vi "AudioTest.Play_Record.vi"(6 "Record Device ID":u32, 7 "Play Device ID":u32=1, 8 "error in (no error)":errorcluster, 9 "Sample Rate (Hz)":dbl, 10 "volume":dbl=40.0 format="%#_13g", 11 "Stimulus Wvfrm":waveform(dbl)(graph)) -> (0 "Error Out":errorcluster, 2 "PlayDur(s)":dbl=1.0 format="%.2p", 3 "Recorded Wvfrm":waveform(dbl)(graph))   [LabVIEW 2018]
uses:
  <vilib>/sound2/lvsound2.llb/Sampling Mode.ctl
  <vilib>/sound2/lvsound2.llb/Sound Data Format.ctl
  Common/Utils/Errors/Error.Error Code List.ctl
  <vilib>/sound2/lvsound2.llb/Sound Output Set Volume (Single).vi
  <vilib>/sound2/lvsound2.llb/Sound Output Write (DBL Single).vi
  <vilib>/sound2/lvsound2.llb/Sound Input Read (DBL).vi
panel:
  in  "Pad Time(s)":dbl=0.25 format="%#_13g"
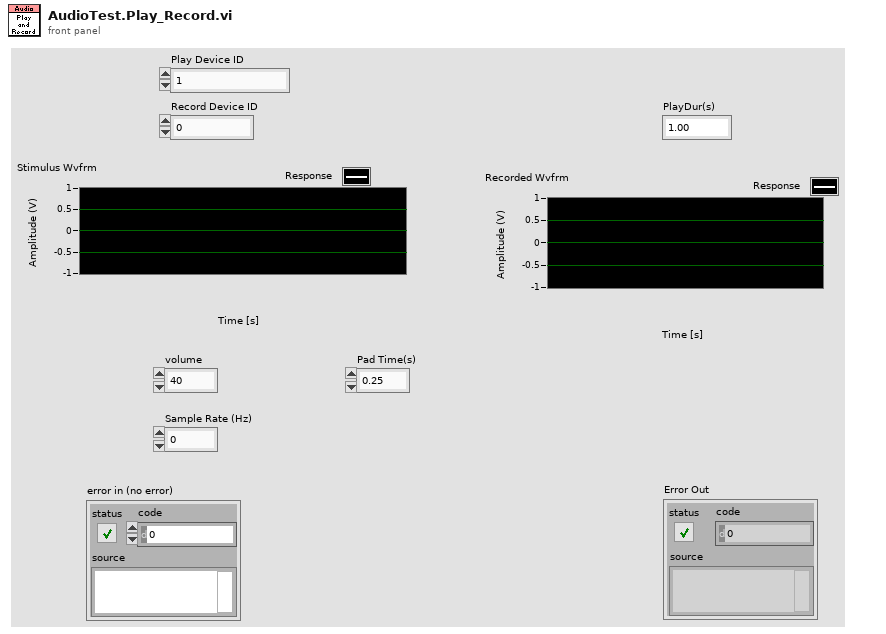
[diagram p1: front panel]
types:
  T1 = typedef "Sound Data Format.ctl" = cluster{"sample rate (S/s)":dbl, "number of channels":i32, "bits per sample":i32}
  T2 = typedef "Error.Error Code List.ctl" = i32
  T3 = typedef "Sampling Mode.ctl" = i32
  T4 = typedef "Sound Output Task ID.ctl" = u32
  T5 = typedef "Sound Input Task ID.ctl" = u32
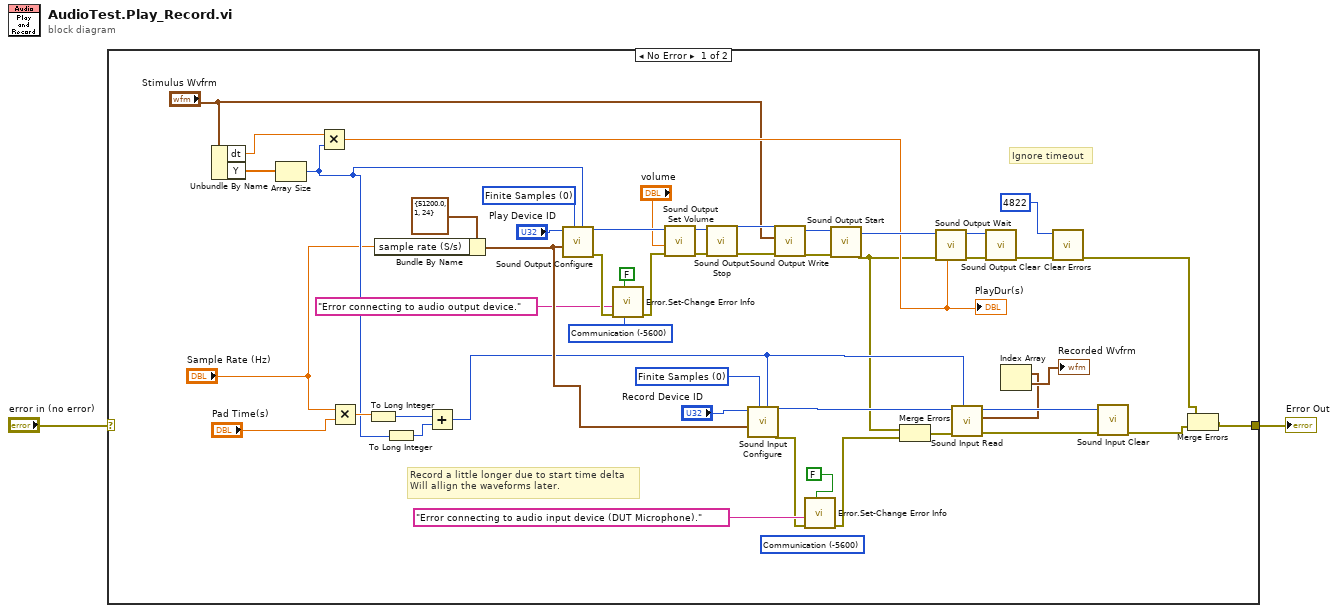
[diagram p0: block diagram]
diagram:
  n1 = case shown="No Error" "error in (no error)" {
    selector: "error in (no error)" -> [_ w52]
    tunnel: [w12 w52] -> w2
    frame No Error {
      (unwired) T2 -5600 items=["No Error"=0, "Abort"=-2, "Misc"=-5000, "Fixture Error"=-5100, "File IO - General"=-5200, "FIle IO - Config Error"=-5201, "Instrument - General"=-5300, "Instrument - Serial Com"=-5301, "Instrument - Camera"=-5302, "Instrument - PS"=-5303, "Instrument - Oscilloscope"=-5304, "Instrument - Function Gen"=-5305, "Instrument - Load"=-5306, "Instrument - Meter"=-5307, "Instrument - Power Control"=-5308, "Instrument - Motion"=-5309, "Instrument - RF"=-5310, "System Exe"=-5400, "Image Processing"=-5500, "Communication"=-5600, "Script - Syntax Error"=-6000, "Script - Invalid Name or Param"=-6100, "Script - Timeout"=-6200, "Invalid Data"=-6300, "FW Update Error"=-6500] ("Std Code")
      w9 = T2 -5600 items=["No Error"=0, "Abort"=-2, "Misc"=-5000, "Fixture Error"=-5100, "File IO - General"=-5200, "FIle IO - Config Error"=-5201, "Instrument - General"=-5300, "Instrument - Serial Com"=-5301, "Instrument - Camera"=-5302, "Instrument - PS"=-5303, "Instrument - Oscilloscope"=-5304, "Instrument - Function Gen"=-5305, "Instrument - Load"=-5306, "Instrument - Meter"=-5307, "Instrument - Power Control"=-5308, "Instrument - Motion"=-5309, "Instrument - RF"=-5310, "System Exe"=-5400, "Image Processing"=-5500, "Communication"=-5600, "Script - Syntax Error"=-6000, "Script - Invalid Name or Param"=-6100, "Script - Timeout"=-6200, "Invalid Data"=-6300, "FW Update Error"=-6500] ("Std Code")
      w46 = T3 0 items=["Finite Samples", "Continuous Samples"] ("sample mode")
      w48 = T3 0 items=["Finite Samples", "Continuous Samples"] ("sample mode")
      # "Ignore timeout"
      # "Record a little longer due to start time delta\nWill allign the waveforms later."
      n2 = Unbundle By Name("Stimulus Wvfrm") -> ("dt"=w22:dbl, "Y"=w39:dbl[])
      n3 = Array Size(array=w39) -> (size(s)=w23:i32)
      n4 = Multiply(x=w22, y=w23) -> (x*y=w21:dbl)
      "PlayDur(s)" <- w21
      n5 = Multiply(x="Sample Rate (Hz)", y="Pad Time(s)") -> (x*y=w37:dbl)
      n6 = To Long Integer(number=w37) -> (32bit integer=w36:i32)
      n7 = Bundle By Name(cluster=T1 {"sample rate (S/s)"=51200.0, "number of channels"=1, "bits per sample"=24} ("sound format"), "sample rate (S/s)"="Sample Rate (Hz)") -> (w40:T1)
      n8 = To Long Integer(number=w23) -> (32bit integer=w35:i32)
      n9 = Add(x=w36, y=w35) -> (x+y=w27:i32)
      n10 = call <vilib>:"Sound Output Configure.vi"("number of samples/ch"=w23, "sample mode"=w48, "sound format"=w40, "device ID"="Play Device ID") -> ("error out"=w11:errorcluster, "task ID"=w51:T4)  [unwired: 6 in]
      n11 = call "Error.Set-Change Error Info.vi"("Std Code"=w9, "Append Details"=FALSE, "error in"=w11, "Description"="Error connecting to audio output device.") -> ("error out"=w10:errorcluster)  [unwired: 7 in]
      n12 = call-poly <vilib>:"Sound Output Set Volume.vi"("error in (no error)"=w10, "volume"="volume", "task ID"=w51) -> ("error out"=w44:errorcluster, "task ID out"=w45:T4)  [unwired: 7 in]
      n13 = call <vilib>:"Sound Output Stop.vi"("error in (no error)"=w44, "task ID"=w45) -> ("error out"=w42:errorcluster, "task ID out"=w43:T4)  [unwired: 8 in]
      n14 = call <vilib>:"Sound Input Configure.vi"("number of samples/ch"=w27, "sample mode"=w46, "sound format"=w40, "device ID"="Record Device ID") -> ("error out"=w6:errorcluster, "task ID"=w26:T5)  [unwired: 6 in]
      n15 = call-poly <vilib>:"Sound Output Write.vi"("error in (no error)"=w42, "data"="Stimulus Wvfrm", "task ID"=w43) -> ("error out"=w28:errorcluster, "task ID out"=w29:T4)  [unwired: 7 in]
      n16 = call "Error.Set-Change Error Info.vi"("Append Details"=FALSE, "error in"=w6, "Description"="Error connecting to audio input device (DUT Microphone).") -> ("error out"=w5:errorcluster)  [unwired: 8 in]
      n17 = call <vilib>:"Sound Output Start.vi"("error in (no error)"=w28, "task ID"=w29) -> ("error out"=w15:errorcluster, "task ID out"=w32:T4)  [unwired: 8 in]
      n18 = Merge Errors(w15, w5) -> (w16:errorcluster)
      n19 = call <vilib>:"Sound Output Wait.vi"("timeout (sec)"=w21, "error in (no error)"=w15, "task ID"=w32) -> ("error out"=w34:errorcluster, "task ID out"=w33:T4)  [unwired: 7 in]
      n20 = call-poly <vilib>:"Sound Input Read.vi"("number of samples/ch"=w27, "error in (no error)"=w16, "task ID"=w26) -> ("error out"=w24:errorcluster, "data"=w19:waveform(dbl)[], "task ID out"=w25:T5)  [unwired: 6 in]
      n21 = call <vilib>:"Sound Output Clear.vi"("error in (no error)"=w34, "task ID"=w33) -> ("error out"=w31:errorcluster)  [unwired: 9 in]
      n22 = Index Array(array=w19) -> (element=→"Recorded Wvfrm":waveform(dbl))  [unwired: 1 in]
      n23 = call <vilib>:"Clear Errors.vi"("error in (no error)"=w31, "specific error code to clear (0: all)"=4822) -> ("error out"=w13:errorcluster)  [unwired: 4 in, 1 out]
      n24 = call <vilib>:"Sound Input Clear.vi"("error in (no error)"=w24, "task ID"=w25) -> ("error out"=w14:errorcluster)  [unwired: 9 in]
      n25 = Merge Errors(w13, w14) -> (w12:errorcluster)
    }
    frame Error {
    }
  }
  "Error Out" <- w2
